vi "Example.vi"(10 "Baud Rate":u32(ring)=57600 items=["75"=75, "110"=110, "134"=134, "150"=150, "300"=300, "600"=600, "1200"=1200, "1800"=1800, "2400"=2400, "4800"=4800, "7200"=7200, "9600"=9600, "14400"=14400, "19200"=19200, "28800"=28800, "38400"=38400, "56000"=56000, "57600"=57600, "115200"=115200, "128000"=128000, "230400"=230400], 11 "Comport":refnum<visa-resource-name>="COM20") -> (0 "error out":errorcluster)   [LabVIEW 2020]
doc: "Initializes the library with a serial comport as the transport method"
uses:
  FirmataClient/Controls/SupportedTransports.ctl
  FirmataClient/.Tmp/Transparent array.ctl
  FirmataClient/Controls/UI-Digital Pin.ctl
  FirmataClient/Controls/UI-PWM Pins.ctl
  FirmataClient/Controls/UI-PWM Pin.ctl
  FirmataClient/Controls/UI-Analog Pins.ctl
  FirmataClient/Controls/UI-Analog Pin.ctl
  FirmataClient/Controls/FirmataPinModes.ctl
panel:
  out "Connected":bool
  out "Firmata Firmware Name":string
  out "Firmata Firmware Version":string
  in  "Stop":bool
  in  "Tab Control":T1(tab)
  in  "Connect":bool
  in  "Connection Details":enum32{"Serial Communication", "Page 2"}(tab)
  in  "Select Transport Mode":T2
  in  "Digital Lines":T3 caption="Digital Lines                             Direction                                         ON/OFF                     Value" {"Pin Value" format="%#_g V"}
  in  "Analog Lines":T5 {"Pin Value" format="%#_g V"}
  in  "PWM / Servo Lines":T7 {"Value" min=0.0 max=10.0 scale=0.0..10.0}
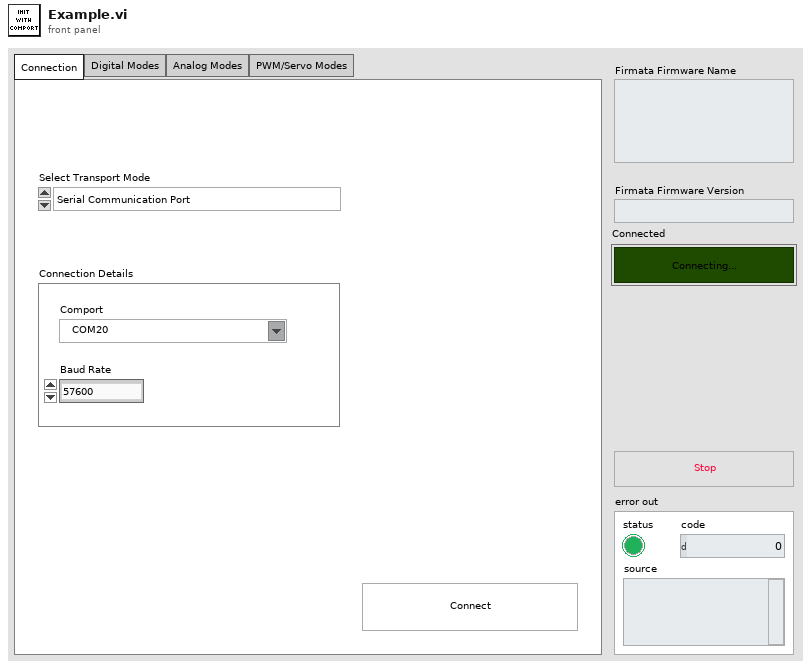
[diagram p1: front panel]
types:
  T1 = enum32{"Connection", "Digital Modes", "Analog Modes", "PWM/Servo Modes"}
  T2 = typedef "SupportedTransports.ctl" = enum16{"Serial Communication Port"}
  T3 = typedef "Transparent array.ctl" = T4[]
  T4 = typedef "UI-Digital Pin.ctl" = cluster{"IO Direction":u16, "Pin Direction":string, "DO Value":u16, "Pin Value":dbl, "Pin Index":string, "Pin Mode":string}
  T5 = typedef "UI-Analog Pins.ctl" = T6[]
  T6 = typedef "UI-Analog Pin.ctl" = cluster{"IO Direction":u16, "Pin Direction":string, "Pin Value":dbl, "Pin Index":string, "Pin Mode":string}
  T7 = typedef "UI-PWM Pins.ctl" = T8[]
  T8 = typedef "UI-PWM Pin.ctl" = cluster{"Pin Mode":u16, "Pin Mode":string, "Value":dbl, "Pin Index":string, "Pin Modes":string}
  T9 = typedef "FirmataPinModes.ctl" = enum16{"DigitalInput", "DigitalOutput", "AnalogInput", "PWM", "Servo", "Shift", "I2C", "OneWire", "Stepper", "Encoder", "Serial", "InputPullup", "Extended.SPI", "Extended.Sonar", "Extended.Tone", "Extended.DHT"}
  T10 = typedef "FirmataPinCapabilitiesAndAnalogMapping.ctl" = cluster{"Supported Modes":T11[], "Analog Channel":u8, "Pin Name":string}
  T11 = typedef "FirmataPinCapability.ctl" = cluster{"PinMode":T9, "Resolution":u8}
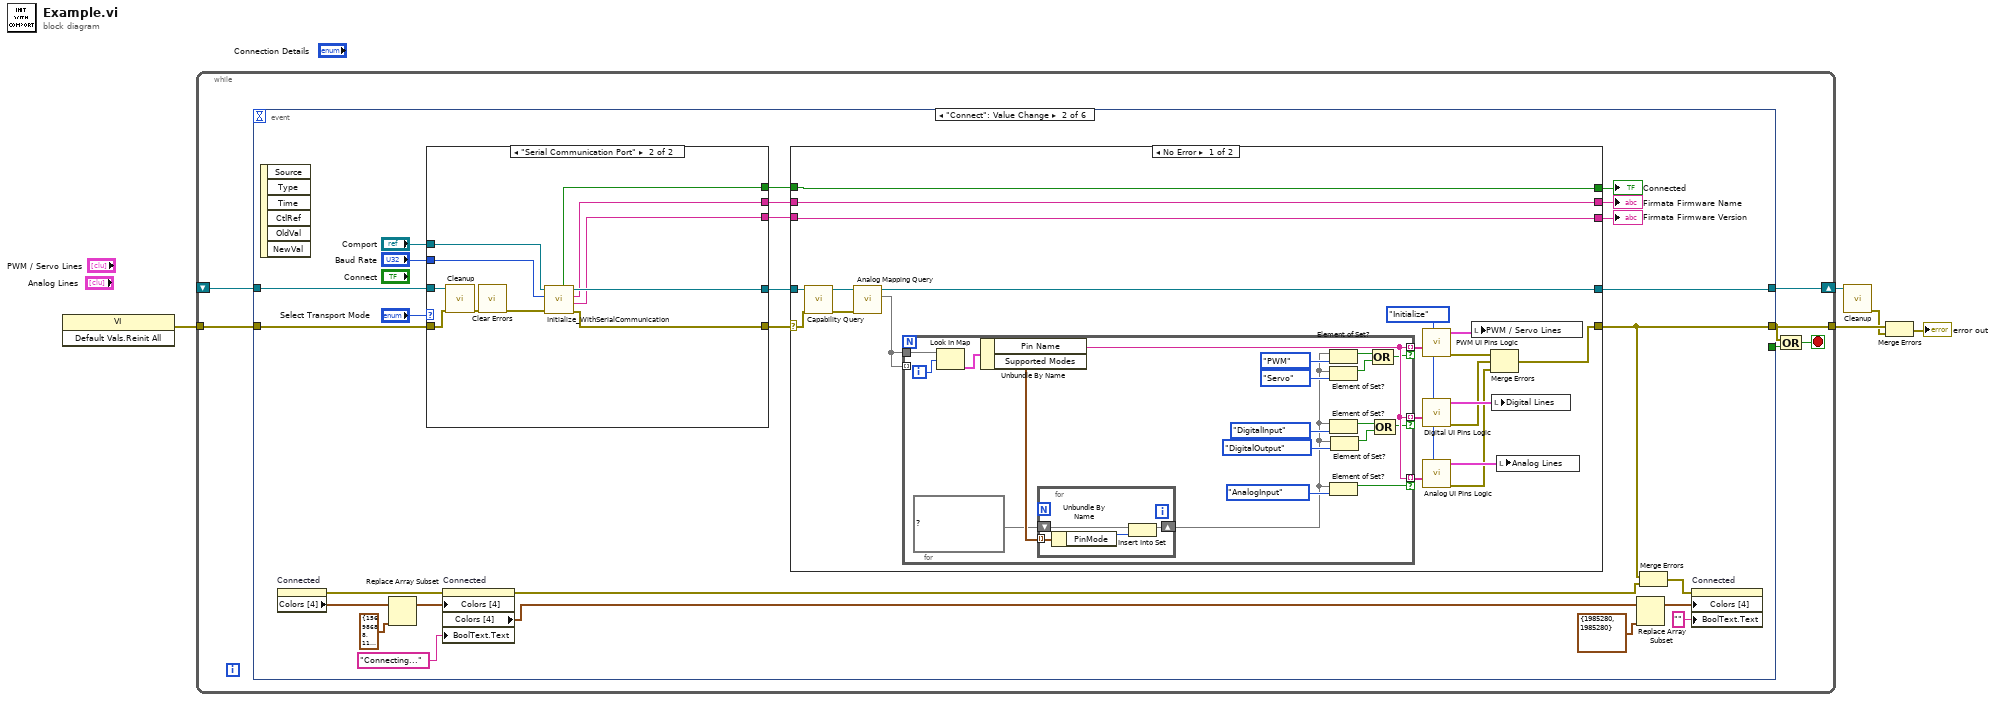
[diagram p0: block diagram]
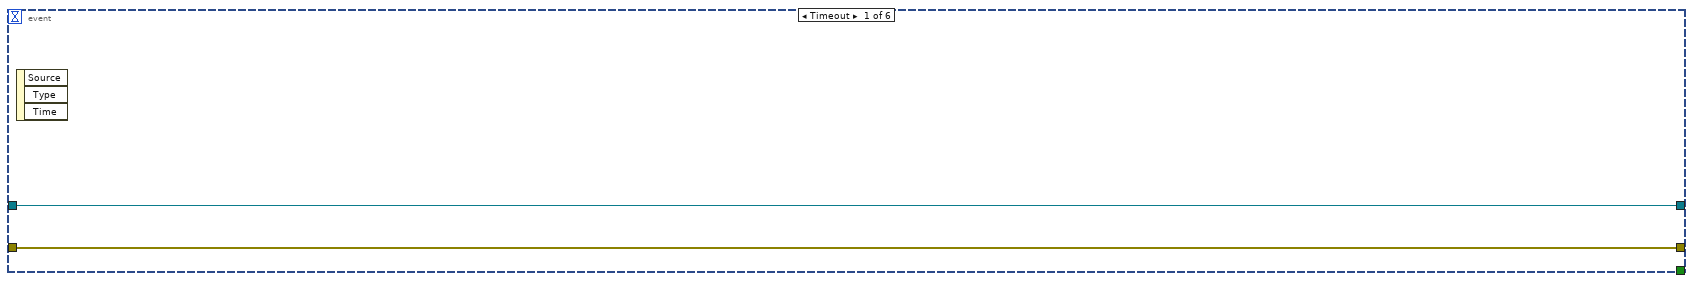
[diagram p2: hidden frame]
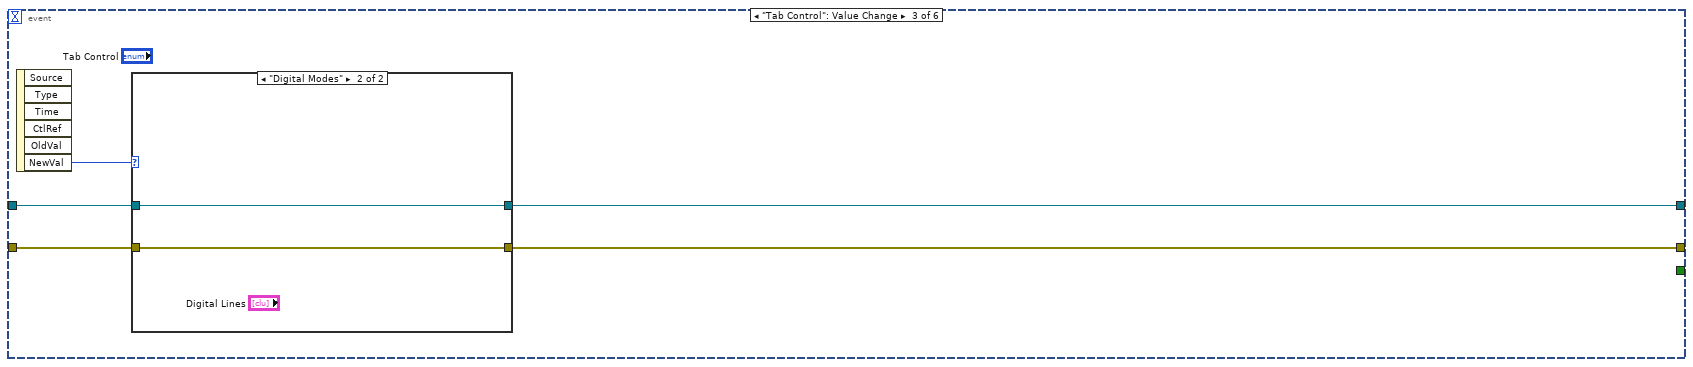
[diagram p5: hidden frame]
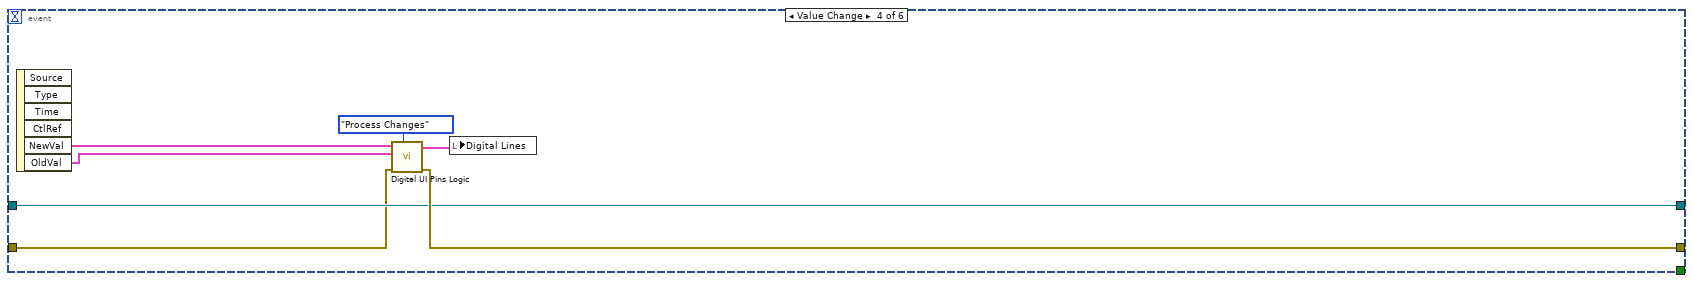
[diagram p7: hidden frame]
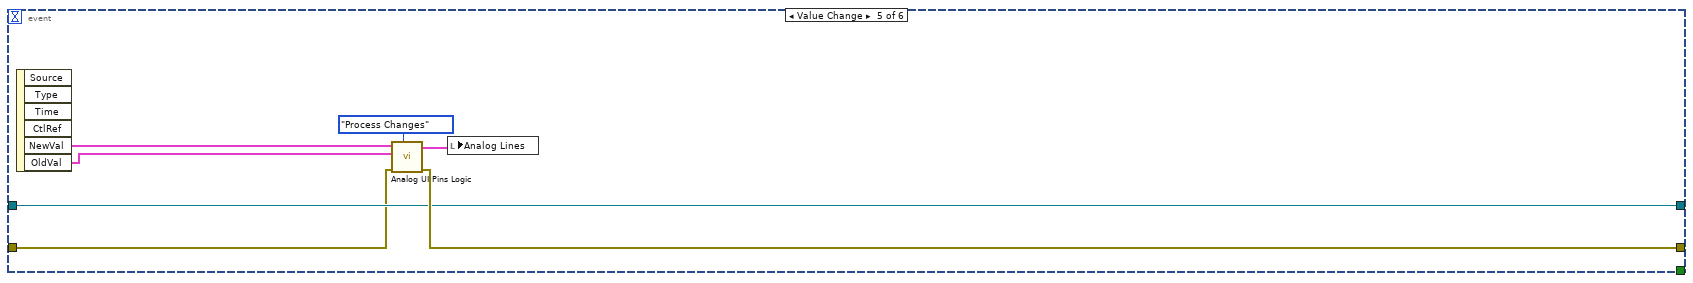
[diagram p8: hidden frame]
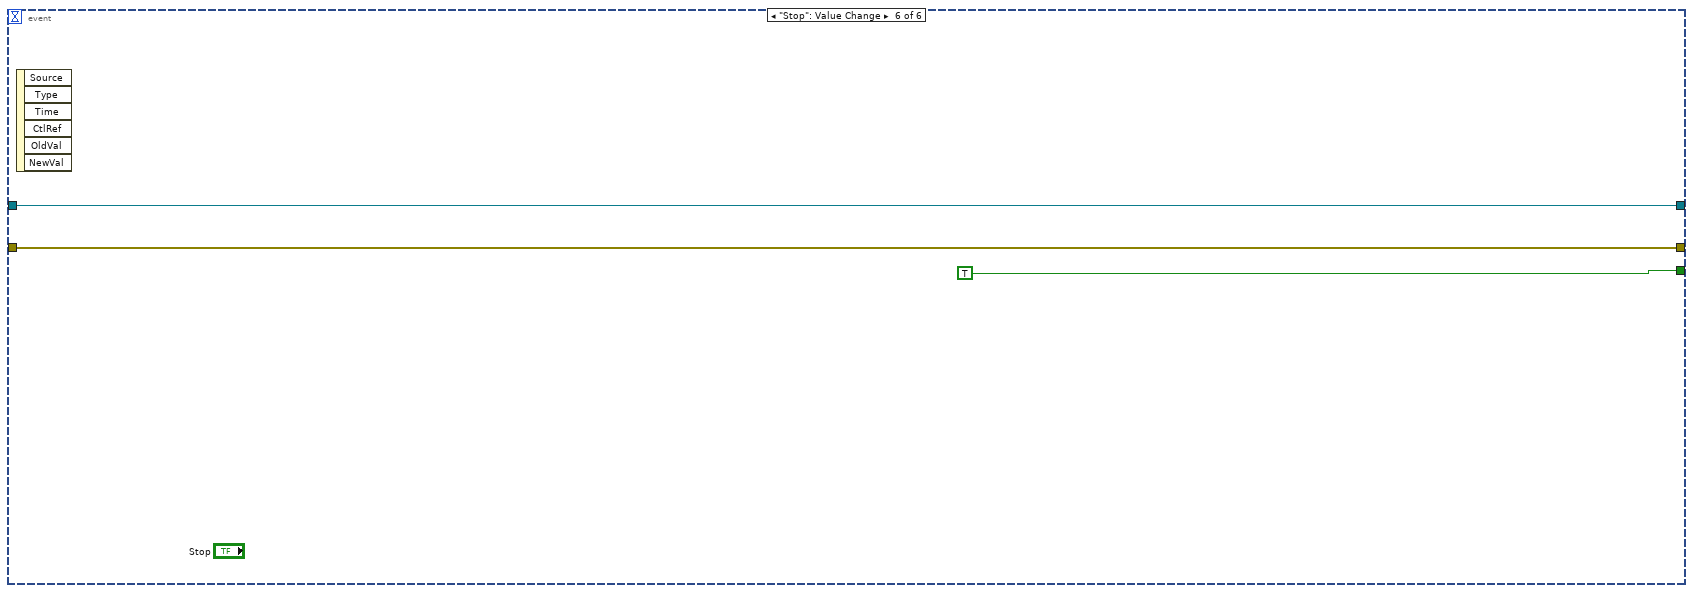
[diagram p9: hidden frame]
diagram:
  n1 = invoke class="VI" method="Default Vals.Reinit All"() -> (error out=w3:errorcluster)  [unwired: 3 in, 2 out]
  n2 = while {
    shift-right: [w11] -> w5
    shift-left: _ -> [w10]
    tunnel: w3 -> [w9]
    tunnel: [w8] -> w2
    stop <- w6 stop-if-true
    n3 = event shown="[1] \"Connect\": Value Change" {
      selector: _ -> [_ _ _ _ _ _]
      dyn-events: _ -> [_ _ _ _ _ _]
      timeout: _ -> [_ _ _ _ _ _]
      tunnel: [_ _ _ _ _ TRUE] -> w7
      tunnel: [w13 w32 w103 w112 w119 w126] -> w11
      tunnel: w10 -> [w13 w37 w102 w112 w119 w126]
      tunnel: [w12 w17 w105 w113 w120 w125] -> w8
      tunnel: w9 -> [w12 w39 w104 w111 w118 w125]
      event Timeout {
        n4 = event-data() -> ()  [unwired: 1 in, 3 out]
      }
      event "Connect": Value Change {
        n5 = event-data() -> ()  [unwired: 1 in, 6 out]
        n6 = property on="Connected" class="Bool (strict)"() -> (error out=w21:errorcluster, "Colors [4]"=w23:cluster{u32, u32}[])  [unwired: 2 in, 1 out]
        n7 = Replace Array Subset(array=w23, new element=cluster{u32, u32} {15698688, 11820800} ("new element/subarray")) -> (w20:cluster{u32, u32}[])  [unwired: 1 in]
        n8 = case shown="\"Serial Communication Port\"" "Select Transport Mode" {
          tunnel: w39 -> [w88 w95]
          tunnel: [w89 w93] -> w33
          tunnel: [w88 w98] -> w34
          tunnel: w37 -> [w89 w97]
          tunnel: "Baud Rate" -> [_ w100]
          tunnel: "Comport" -> [_ w99]
          tunnel: [_ w92] -> w31
          tunnel: [_ w91] -> w30
          tunnel: [_ w90] -> w29
          frame Default {
          }
          frame "Serial Communication Port" {
            n9 = call "Cleanup.vi"("error in"=w95, "Refnum In"=w97) -> ("error out"=w96:errorcluster)  [unwired: 8 in, 1 out]
            n10 = call <vilib>:"Clear Errors.vi"("error in (no error)"=w96) -> ("error out"=w94:errorcluster)  [unwired: 5 in, 1 out]
            n11 = call "Initialize_WithSerialCommunication.vi"("error in"=w94, "Baud Rate"=w100, "Comport"=w99) -> ("error out"=w98:errorcluster, "FirmataFirmwareVersion"=w91:string, "FirmataFirmwareName"=w90:string, "Refnum Out"=w93:refnum<vi>, "Connected"=w92:bool)  [unwired: 4 in]
          }
        }
        n12 = property on="Connected" class="Bool (strict)"(error in=w21, "Colors [4]"=w20, "BoolText.Text"="Connecting..." ("Boolean Text.Text")) -> (error out=w16:errorcluster, "Colors [4]"=w18:cluster{u32, u32}[])  [unwired: 1 in, 1 out]
        n13 = case shown="No Error" w34 {
          selector: w34 -> [w54 w87]
          tunnel: [w49 w87] -> w17
          tunnel: [w59 w86] -> w32
          tunnel: w33 -> [w55 w86]
          tunnel: w31 -> [w48 w83]
          tunnel: w30 -> [w46 w85]
          tunnel: w29 -> [w47 w84]
          tunnel: [w48 w83] -> w28
          tunnel: [w47 w84] -> w27
          tunnel: [w46 w85] -> w26
          frame No Error {
            w44 = enum16{"Initialize", "Process Changes"}."Initialize" ("Mode")
            n14 = call "Capability Query.vi"("error in (no error)"=w54, "Refnum In"=w55) -> ("error out"=w57:errorcluster, "Refnum Out"=w56:refnum<vi>)  [unwired: 7 in, 1 out]
            n15 = call "Analog Mapping Query.vi"("error in (no error)"=w57, "Refnum In"=w56) -> ("Board Capabilities"=w53:map{i32, T10}, "Refnum Out"=w59:refnum<vi>)  [unwired: 7 in, 1 out]
            n16 = for {
              tunnel: w53 -> [w78]
              tunnel: w53 -> [_] mode=indexing
              tunnel: [w73] -> w42 mode=indexing if=w62
              tunnel: [w73] -> w41 mode=indexing if=w61
              tunnel: [w73] -> w40 mode=indexing if=w60
              i -> [w77]
              n17 = Look In Map(map=w78, key=w77) -> (value=w76:T10)  [unwired: 1 in, 1 out]
              n18 = Unbundle By Name(w76) -> ("Pin Name"=w73:string, "Supported Modes"=w75:T11[])
              n19 = for {
                tunnel: w75 -> [w82] mode=indexing
                shift-right: [w79] -> w65
                shift-left: set{T9} {} ("set in") -> [w80]
                n20 = Unbundle By Name(w82) -> ("PinMode"=w81:T9)
                n21 = Insert Into Set(10:w81, 11:w80) -> (3:w79:set{T9})  [unwired: 1 out]
              }
              n22 = Element of Set?(10:FirmataPinModes."PWM" ("element"), 11:w65) -> (3:w63:bool)
              n23 = Element of Set?(10:FirmataPinModes."Servo" ("element"), 11:w65) -> (3:w64:bool)
              n24 = Element of Set?(10:FirmataPinModes."DigitalInput" ("element"), 11:w65) -> (3:w67:bool)
              n25 = Element of Set?(10:FirmataPinModes."AnalogInput" ("element"), 11:w65) -> (3:w60:bool)
              n26 = Element of Set?(10:FirmataPinModes."DigitalOutput" ("element"), 11:w65) -> (3:w68:bool)
              n27 = Compound Arithmetic op=OR(w63, w64) -> (w62:bool)
              n28 = Compound Arithmetic op=OR(w67, w68) -> (w61:bool)
            }
            n29 = call "PWM UI Pins Logic.vi"("Mode"=w44, "Initial Pin Names"=w42) -> ("error out"=w51:errorcluster, "Updated Value"=w58:T7)  [unwired: 8 in]
            n30 = call "Digital UI Pins Logic.vi"("Mode"=w44, "Initial Pin Names"=w41) -> ("error out"=w50:errorcluster, "Updated Value"=w52:T3)  [unwired: 8 in]
            n31 = call "Analog UI Pins Logic.vi"("Mode"=w44, "Initial Pin Names"=w40) -> ("error out"=w43:errorcluster, "Updated Value"=w45:T5)  [unwired: 8 in]
            n32 = local write "PWM / Servo Lines"(w58) -> ()
            n33 = Merge Errors(w51, w50, w43) -> (w49:errorcluster)
            n34 = local write "Digital Lines"(w52) -> ()
            n35 = local write "Analog Lines"(w45) -> ()
          }
          frame Error {
          }
        }
        "Firmata Firmware Name" <- w27
        "Firmata Firmware Version" <- w26
        "Connected" <- w28
        n36 = Replace Array Subset(array=w18, new element=cluster{"Numeric":u32, "Numeric":u32} {"Numeric"=1985280, "Numeric"=1985280} ("element")) -> (w25:cluster{u32, u32}[])  [unwired: 1 in]
        n37 = Merge Errors(w17, w16) -> (w15:errorcluster)
        n38 = property on="Connected" class="Bool (strict)"(error in=w15, "Colors [4]"=w25, "BoolText.Text"="" ("Boolean Text.Text")) -> ()  [unwired: 1 in, 2 out]
      }
      event "Tab Control": Value Change {
        n39 = event-data() -> ("NewVal"=w101:T1)  [unwired: 1 in, 5 out]
        n40 = case shown="\"Digital Modes\"" w101 {
          tunnel: [w107 w109] -> w105
          tunnel: w104 -> [w107 w109]
          tunnel: [w106 w108] -> w103
          tunnel: w102 -> [w106 w108]
          frame "Connection", Default {
          }
          frame "Digital Modes" {
          }
        }
      }
      event Value Change {
        n41 = event-data() -> ("NewVal"=w116:T3, "OldVal"=w115:T3)  [unwired: 1 in, 4 out]
        n42 = call "Digital UI Pins Logic.vi"("Mode"=enum16{"Initialize", "Process Changes"}."Process Changes", "error in"=w111, "OldVal"=w115, "NewVal"=w116) -> ("error out"=w113:errorcluster, "Updated Value"=w114:T3)  [unwired: 6 in]
        n43 = local write "Digital Lines"(w114) -> ()
      }
      event Value Change {
        n44 = event-data() -> ("NewVal"=w123:T5, "OldVal"=w122:T5)  [unwired: 1 in, 4 out]
        n45 = call "Analog UI Pins Logic.vi"("Mode"=enum16{"Initialize", "Process Changes"}."Process Changes", "error in"=w118, "OldVal"=w122, "NewVal"=w123) -> ("error out"=w120:errorcluster, "Updated Value"=w121:T5)  [unwired: 6 in]
        n46 = local write "Analog Lines"(w121) -> ()
      }
      event "Stop": Value Change {
        n47 = event-data() -> ()  [unwired: 1 in, 6 out]
      }
    }
    n48 = Compound Arithmetic op=OR(w8, w7) -> (w6:bool)
  }
  n49 = call "Cleanup.vi"("Refnum In"=w5) -> ("error out"=w1:errorcluster)  [unwired: 9 in, 1 out]
  n50 = Merge Errors(w2, w1) -> (→"error out":errorcluster)
